vi "Exposure.vi"(0 "Command":T1(ring), 1 "Exposure Time":dbl) -> (2 "Error":bool, 3 "float":dbl, 4 "integer":i32)   [LabVIEW 2014]
panel:
  # "seconds"
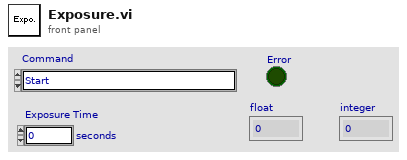
[diagram p1: front panel]
types:
  T1 = enum16{"Start", "Stop", "Abort", "Pause", "SetExposureTime", "GetExposureTimeRemaining", "Resume", "Readout", "GetExposureTime", "GetTotalPixels", "GetPixelsRemaining"}
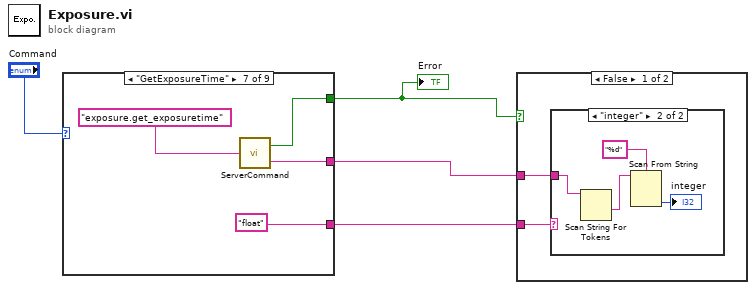
[diagram p0: block diagram]
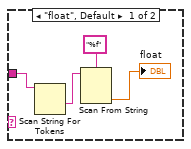
[diagram p2: hidden frame]
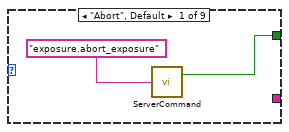
[diagram p4: hidden frame]
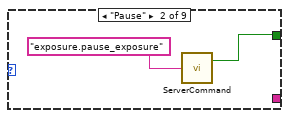
[diagram p5: hidden frame]
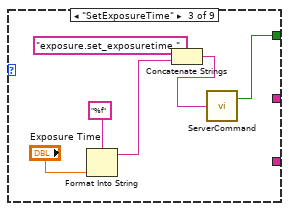
[diagram p6: hidden frame]
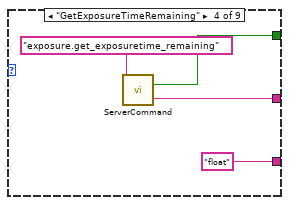
[diagram p7: hidden frame]
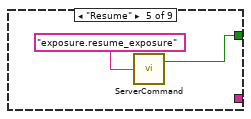
[diagram p8: hidden frame]
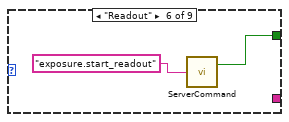
[diagram p9: hidden frame]
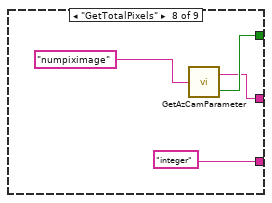
[diagram p10: hidden frame]
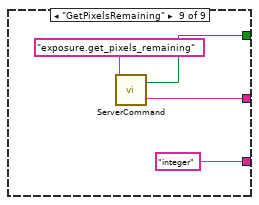
[diagram p11: hidden frame]
diagram:
  n1 = case shown="\"GetExposureTime\"" "Command" {
    tunnel: [_ _ _ w16 _ _ w23 w27 w32] -> w1
    tunnel: [_ _ _ "float" _ _ "float" "integer" "integer"] -> w3
    tunnel: [w6 w7 w9 w15 w19 w22 w24 w28 w31] -> w2
    frame "Abort", Default {
      n2 = call "ServerCommand.vi"("Command"="exposure.abort_exposure") -> ("Error"=w6:bool)  [unwired: 1 out]
    }
    frame "Pause" {
      n3 = call "ServerCommand.vi"("Command"="exposure.pause_exposure") -> ("Error"=w7:bool)  [unwired: 1 out]
    }
    frame "SetExposureTime" {
      n4 = Format Into String(format string="%f", "Exposure Time") -> (resulting string=w11:string)  [unwired: 2 in, 1 out]
      n5 = Concatenate Strings("exposure.set_exposuretime ", w11) -> (w10:string)
      n6 = call "ServerCommand.vi"("Command"=w10) -> ("Error"=w9:bool)  [unwired: 1 out]
    }
    frame "GetExposureTimeRemaining" {
      n7 = call "ServerCommand.vi"("Command"="exposure.get_exposuretime_remaining") -> ("Error"=w15:bool, "Reply"=w16:string)
    }
    frame "Resume" {
      n8 = call "ServerCommand.vi"("Command"="exposure.resume_exposure") -> ("Error"=w19:bool)  [unwired: 1 out]
    }
    frame "Readout" {
      n9 = call "ServerCommand.vi"("Command"="exposure.start_readout") -> ("Error"=w22:bool)  [unwired: 1 out]
    }
    frame "GetExposureTime" {
      n10 = call "ServerCommand.vi"("Command"="exposure.get_exposuretime") -> ("Error"=w24:bool, "Reply"=w23:string)
    }
    frame "GetTotalPixels" {
      n11 = call "GetAzCamParameter.vi"("Parameter"="numpiximage") -> ("Error"=w28:bool, "Value"=w27:string)
    }
    frame "GetPixelsRemaining" {
      n12 = call "ServerCommand.vi"("Command"="exposure.get_pixels_remaining") -> ("Error"=w31:bool, "Reply"=w32:string)
    }
  }
  "Error" <- w2
  n13 = case shown="False" w2 {
    tunnel: w3 -> [w36 _]
    tunnel: w1 -> [w35 _]
    frame False {
      n14 = case shown="\"integer\"" w36 {
        tunnel: w35 -> [w38 w42]
        frame "float", Default {
          n15 = Scan String For Tokens(9:w38) -> (1:w37:string)  [unwired: 5 in, 3 out]
          n16 = Scan From String(format string="%f", input string=w37) -> (output 1=→"float":dbl)  [unwired: 3 in, 3 out]
        }
        frame "integer" {
          n17 = Scan String For Tokens(9:w42) -> (1:w41:string)  [unwired: 5 in, 3 out]
          n18 = Scan From String(format string="%d", input string=w41) -> (output 1=→"integer":i32)  [unwired: 3 in, 3 out]
        }
      }
    }
    frame True {
    }
  }
